vi "waitforpump.vi"(0 "object in":refnum<class "Application.lvclass">=refnum, 2 "Timeout(s)":dbl=60.0 caption="Timeout (s)", 5 "error in (no error)":errorcluster) -> (14 "object out":refnum<class "Application.lvclass">, 16 "Timeout":bool=TRUE, 19 "error out":errorcluster)   [LabVIEW 2021, in "Application.lvclass"]
uses:
  Application.lvclass
  Hamamatsu_class/Hamamatsu.lvclass
  AD2_SDK_class/AD2_SDK.lvclass
  Valve_class/Valve.lvclass
  Ismatec_class/Ismatec.lvclass
  ExperimentSeries_class/ExperimentSeries.lvclass
  CetoniPump_class/CetoniPump.lvclass
  Prior_Zmotor_class/Prior_Zmotor.lvclass
  ExperimentSeries2_class/ExperimentSeries2.lvclass
  Application.lvclass/Application.ctl
panel:
  out "Elapsed Time (s)":dbl=1.0003447532653809
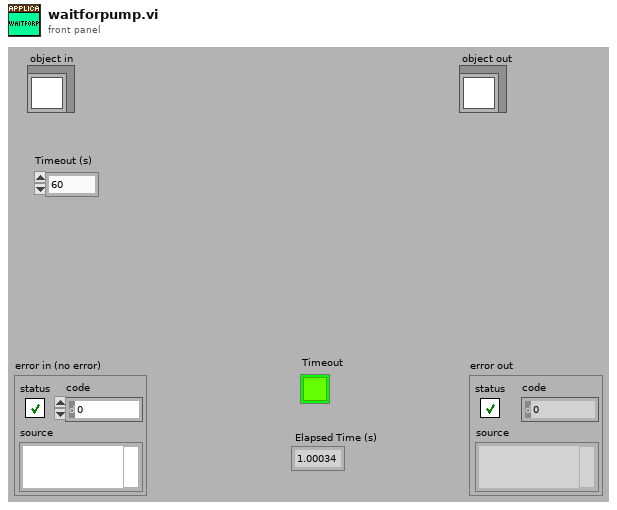
[diagram p1: front panel]
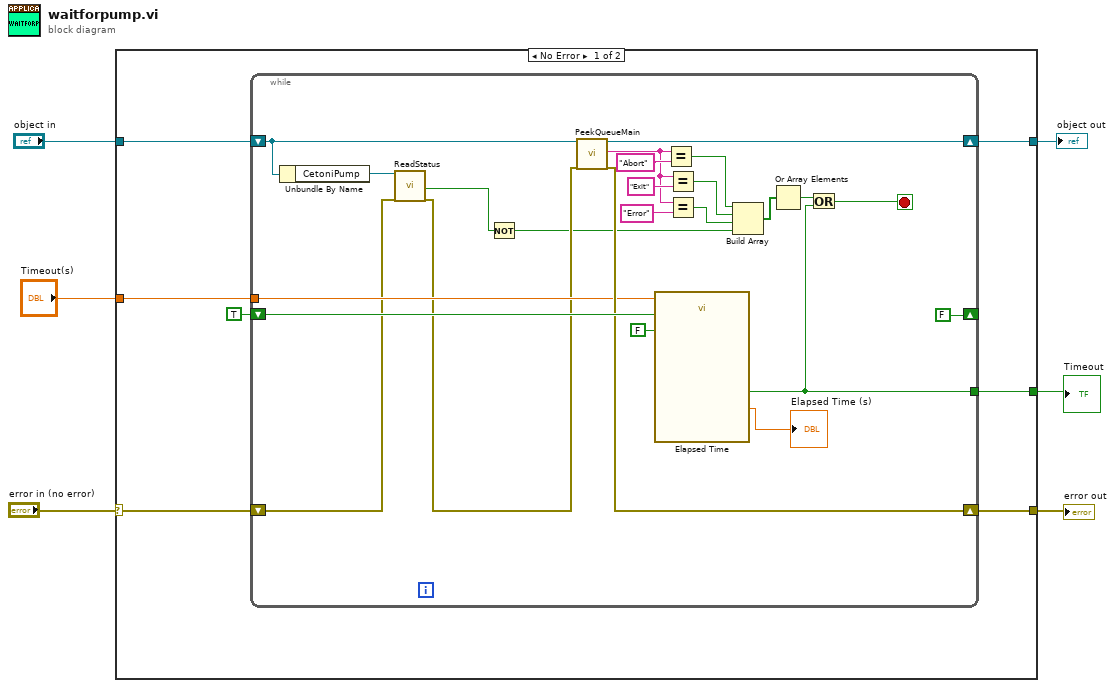
[diagram p0: block diagram]
diagram:
  n1 = case shown="No Error" "error in (no error)" {
    selector: "error in (no error)" -> [w8 w39]
    tunnel: [w7 w39] -> w5
    tunnel: [w13 w38] -> w3
    tunnel: "object in" -> [w12 w38]
    tunnel: "Timeout(s)" -> [w11 _]
    tunnel: [w9 _] -> w1
    frame No Error {
      n2 = while {
        shift-right: [w37] -> w13
        shift-left: w12 -> [w19]
        shift-right: [FALSE] -> _
        shift-left: TRUE -> [w26]
        shift-right: [w23] -> w7
        shift-left: w8 -> [w17]
        tunnel: w11 -> [w21]
        tunnel: [w20] -> w9
        stop <- w27 stop-if-true
        n3 = Unbundle By Name(w19) -> ("CetoniPump"=w18:refnum<class "CetoniPump.lvclass">)
        n4 = call-dynamic "ReadStatus.vi"("object in"=w18, "error in (no error)"=w17) -> ("Is pumping"=w15:bool, "error out"=w16:errorcluster)  [unwired: 13 in, 3 out]
        n5 = Not(x=w15) -> (.not. x?=w14:bool)
        n6 = call-dynamic "PeekQueueMain.vi"("object in"=w19, "error in (no error)"=w16) -> ("object out"=w37:refnum<class "Application.lvclass">, "Message"=w29:string, "error out"=w23:errorcluster)  [unwired: 14 in, 1 out]
        n7 = call "Elapsed Time"("Time Target (s)"=w21, "Reset"=w26, "Auto Reset"=FALSE) -> ("Elapsed Time (s)"=→"Elapsed Time (s)":dbl, "Time has Elapsed"=w20:bool)  [unwired: 9 in, 6 out]
        n8 = Equal?(x=w29, y="Abort") -> (x = y?=w32:bool)
        n9 = Equal?(x=w29, y="Exit") -> (x = y?=w31:bool)
        n10 = Equal?(x=w29, y="Error") -> (x = y?=w33:bool)
        n11 = Build Array(w32, w31, w33, w14) -> (w30:bool[])
        n12 = Or Array Elements(Boolean array=w30) -> (logical OR=w28:bool)
        n13 = Or(x=w28, y=w20) -> (x .or. y?=w27:bool)
      }
    }
    frame Error {
    }
  }
  "error out" <- w5
  "object out" <- w3
  "Timeout" <- w1
